vi "PDF_Generator.vi"(7 "all rows":string[][](array[string]), 8 "error in (no error)":errorcluster, 9 "PDF folder Path":path=path "C:/Users/A. Halstesd Evander/Downloads", 10 "Filename":string="12345", 11 "module path":path=path "C:/Users/A. Halstesd Evander/Documents/VCU_BoxBuild/SourceCode/CSVConversion.py") -> (0 "error out":errorcluster)   [LabVIEW 2024, in "Test_2.lvlib"]
uses:
  Test_2.lvlib
panel:
  out "return value":string
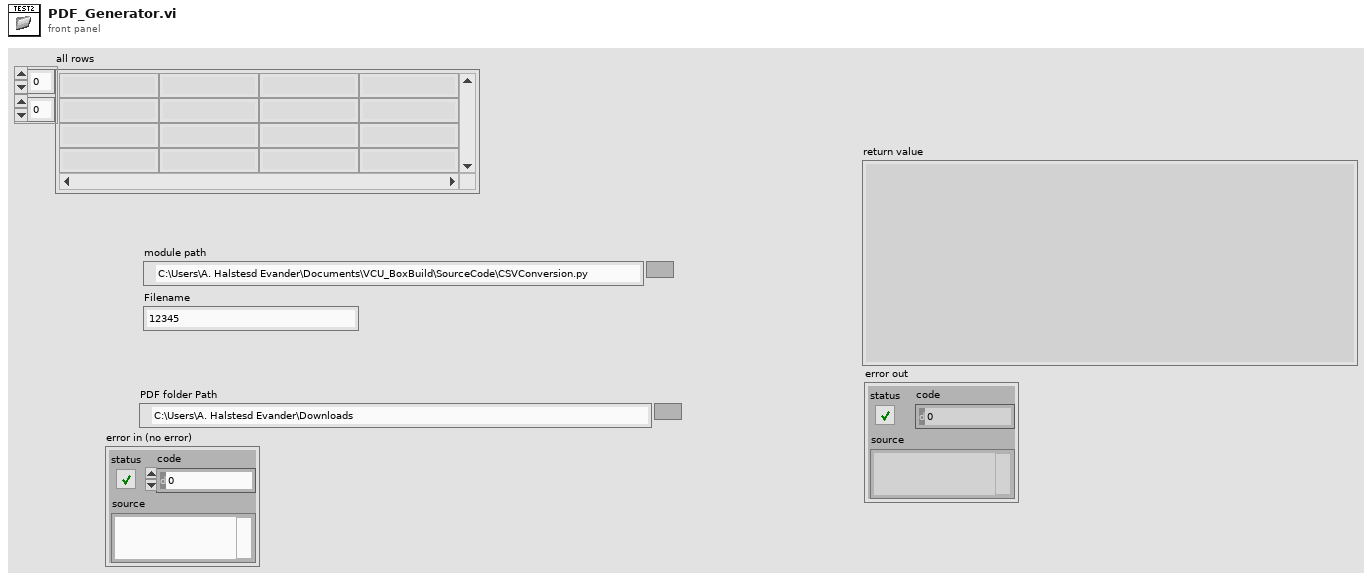
[diagram p1: front panel]
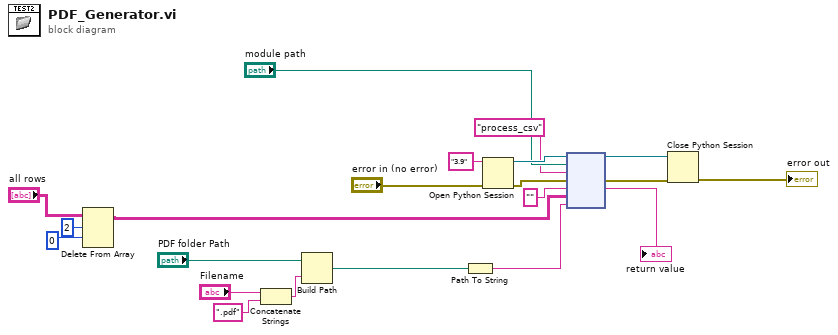
[diagram p0: block diagram]
diagram:
  n1 = Delete From Array(array="all rows", length=2, index (row)=0) -> (array with subset deleted=w1:string[][])  [unwired: 1 in, 1 out]
  n2 = Concatenate Strings("Filename", ".pdf" ("string")) -> (w9:string)
  n3 = Build Path(base path="PDF folder Path", name or relative path=w9) -> (appended path=w14:path)
  n4 = Path To String(path=w14) -> (string=w5:string)
  n5 = Open Python Session(python version="3.9" ("Python version"), 3:"error in (no error)") -> (session out=w20:refnum<k35>, error out=w19:errorcluster)  [unwired: 1 in]
  n6 = node(w20, "module path", "process_csv" ("function name"), w19, "", w1, w5) -> (w11:refnum<k35>, w12:errorcluster, →"return value":string)  [unwired: 2 in, 2 out]
  n7 = Close Python Session(session in=w11, error in=w12) -> (11:→"error out":errorcluster)
